vi "ValidateValue.vi"(10 "SEQ 1":cluster{dbl, dbl, dbl}(slide) scale=0.0..20.0 scale format="%#.1g", 11 "Slide Refnum in":refnum<vi>) -> (2 "SEQ out":cluster{dbl, dbl, dbl}(slide) scale=0.0..20.0 scale format="%#.1g", 3 "Slide Refnum out":refnum<vi>)   [LabVIEW 2012, in "Time Slider.xctl"]
uses:
  Time Slider.xctl
panel:
  # "Check if slider values are in order"
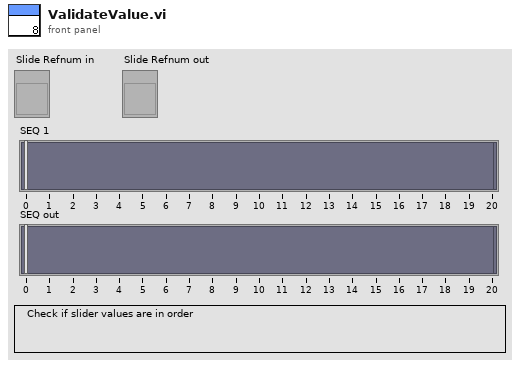
[diagram p1: front panel]
types:
  T1 = cluster{"Scale.Maximum":dbl, "Scale.Maximum":dbl, "Scale.Maximum":dbl}
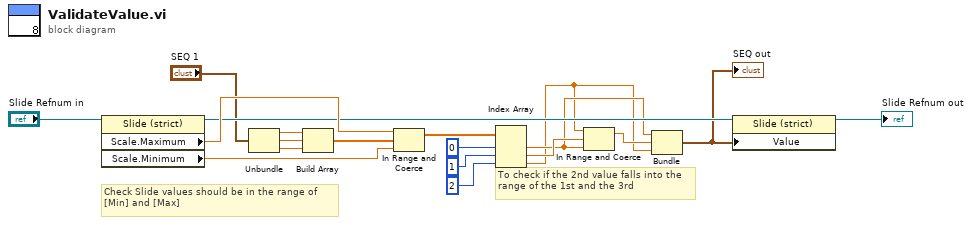
[diagram p0: block diagram]
diagram:
  # "To check if the 2nd value falls into the range of the 1st and the 3rd"
  # "Check Slide values should be in the range of [Min] and [Max]"
  n1 = property class="Slide (strict)"(reference="Slide Refnum in") -> (reference out=w7:refnum<vi>, "Scale.Maximum"=w10:dbl, "Scale.Minimum"=w9:dbl)  [unwired: 1 in, 1 out]
  n2 = Unbundle("SEQ 1") -> (w19:dbl, w18:dbl, w17:dbl)
  n3 = Build Array(w19, w18, w17) -> (w16:dbl[])
  n4 = In Range and Coerce(upper limit=w10, x=w16, lower limit=w9) -> (coerced(x)=w15:dbl[])  [unwired: 1 out]
  n5 = Index Array(array=w15, index #1=0, index #2=1, index #3=2) -> (element #1=w5:dbl, element #2=w8:dbl, element #3=w4:dbl)
  n6 = In Range and Coerce(upper limit=w4, x=w8, lower limit=w5) -> (coerced(x)=w6:dbl)  [unwired: 1 out]
  n7 = Bundle("Scale.Maximum"=w5, "Scale.Maximum"=w6, "Scale.Maximum"=w4) -> (w2:T1)  [unwired: 1 in]
  "SEQ out" <- w2
  n8 = property class="Slide (strict)"(reference=w7, "Value"=w2) -> (reference out=→"Slide Refnum out":refnum<vi>)  [unwired: 1 in, 1 out]
